vi "Get_YPRHfH.vi"(5 "Device Number":T1, 7 "Update":bool) -> (2 "YRPHfH":T2)   [LabVIEW 2016]
doc: "This navX VI returns the Yaw, Roll, Pitch, Heading, Fused Heading of the navX."
uses:
  _TypeDefs/FRIC_navX_DeviceNumbersTypeDef.ctl
  _TypeDefs/Z900_navX_DeviceRegisters.ctl
  _Util/Z900_navX_Util_LittleEndian_to_BigEndian.vi
  _Internal/FRIC_navX_Get_Registry.vi
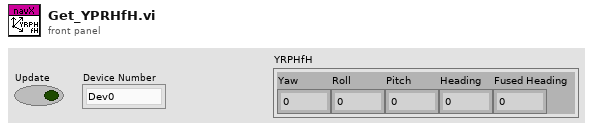
[diagram p1: front panel]
types:
  T1 = typedef "FRIC_navX_DeviceNumbersTypeDef.ctl" = enum16{"Dev0", "Dev1", "Dev2", "Dev3"}
  T2 = cluster{"Yaw":dbl, "Roll":dbl, "Pitch":dbl, "Heading":dbl, "Fused Heading":dbl}
  T3 = typedef "Z900_navX_DeviceRegisters.ctl" = u8
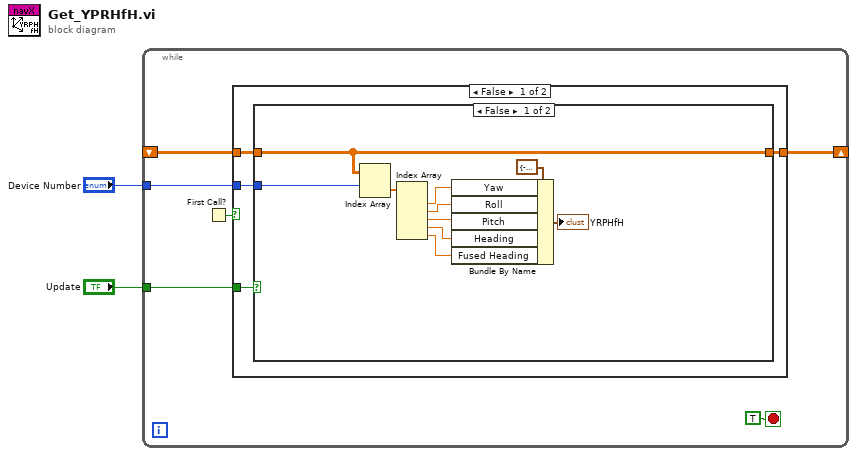
[diagram p0: block diagram]
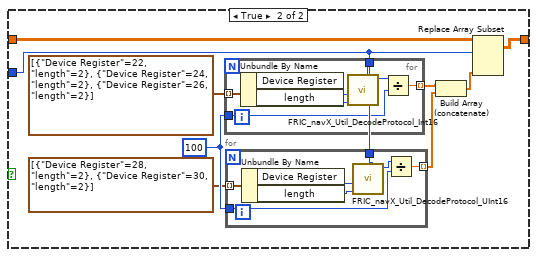
[diagram p2: hidden frame]
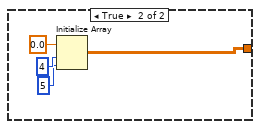
[diagram p3: hidden frame]
diagram:
  n1 = while {
    shift-right: [w6] -> _
    shift-left: _ -> [w7]
    tunnel: "Update" -> [w5]
    tunnel: "Device Number" -> [w4]
    stop <- TRUE stop-if-true
    n2 = First Call?() -> (First Call?: T/F=w3:bool)
    n3 = case shown="False" w3 {
      tunnel: w7 -> [w12 _]
      tunnel: [w11 w49] -> w6
      tunnel: w5 -> [w9 _]
      tunnel: w4 -> [w10 _]
      frame False {
        n4 = case shown="False" w9 {
          tunnel: [w22 w29] -> w11
          tunnel: w12 -> [w22 w31]
          tunnel: w10 -> [w21 w30]
          frame False {
            n5 = Index Array(array=w22, index (row)=w21) -> (element=w18:dbl[])  [unwired: 1 in]
            n6 = Index Array(array=w18) -> (element #1=w17:dbl, element #2=w16:dbl, element #3=w15:dbl, element #4=w14:dbl, element #5=w13:dbl)  [unwired: 5 in]
            n7 = Bundle By Name(cluster=T2 {"Yaw"=-0.34, "Roll"=0.2, "Pitch"=0.2, "Heading"=0.0, "Fused Heading"=359.65} ("YRPHfH"), "Yaw"=w17, "Roll"=w16, "Pitch"=w15, "Heading"=w14, "Fused Heading"=w13) -> (→"YRPHfH":T2)
          }
          frame True {
            w27 = 100 ("y")
            n8 = for {
              tunnel: w30 -> [w37]
              tunnel: cluster{"Device Register":T3, "length":i32}[] [{"Device Register"=22, "length"=2}, {"Device Register"=24, "length"=2}, {"Device Register"=26, "length"=2}] ("Array") -> [w36] mode=indexing
              tunnel: w27 -> [w33]
              tunnel: [w32] -> w25 mode=indexing
              n9 = Unbundle By Name(w36) -> ("Device Register"=w35:T3, "length"=w38:i32)
              n10 = call "FRIC_navX_Util_DecodeProtocol_Int16.vi"("Device Number"=w37, "length"=w38, "Device Register"=w35) -> ("Value"=w34:i16)  [unwired: 8 in]
              n11 = Divide(x=w34, y=w33) -> (x/y=w32:dbl)
            }
            n12 = for {
              tunnel: cluster{"Device Register":T3, "length":i32}[] [{"Device Register"=28, "length"=2}, {"Device Register"=30, "length"=2}] ("Array") -> [w45] mode=indexing
              tunnel: w30 -> [w42]
              tunnel: w27 -> [w40]
              tunnel: [w39] -> w24 mode=indexing
              n13 = Unbundle By Name(w45) -> ("Device Register"=w44:T3, "length"=w43:i32)
              n14 = call "FRIC_navX_Util_DecodeProtocol_UInt16.vi"("Device Number"=w42, "length"=w43, "Device Register"=w44) -> ("Value"=w41:u16)  [unwired: 8 in]
              n15 = Divide(x=w41, y=w40) -> (x/y=w39:dbl)
            }
            n16 = Build Array (concatenate)(w25, w24) -> (w23:dbl[])
            n17 = Replace Array Subset(array=w31, new element=w23, index (row)=w30) -> (w29:dbl[][])  [unwired: 1 in]
          }
        }
      }
      frame True {
        n18 = Initialize Array(0.0, 4, 5 ("dimension size")) -> (w49:dbl[][])
      }
    }
  }
